vi "XBOX_Joystick_Name.vi"(9 "POVs":i16[](array[numeric]), 10 "Buttons":bool[](array[boolean]), 11 "Axes":dbl[](array[numeric])) -> (2 "Named Axes":T1, 3 "Named Buttons":T2)   [LabVIEW 2018]
uses:
  TypeDefs/XBoxButtons_Type.ctl
  TypeDefs/XBoxAxes_Type.ctl
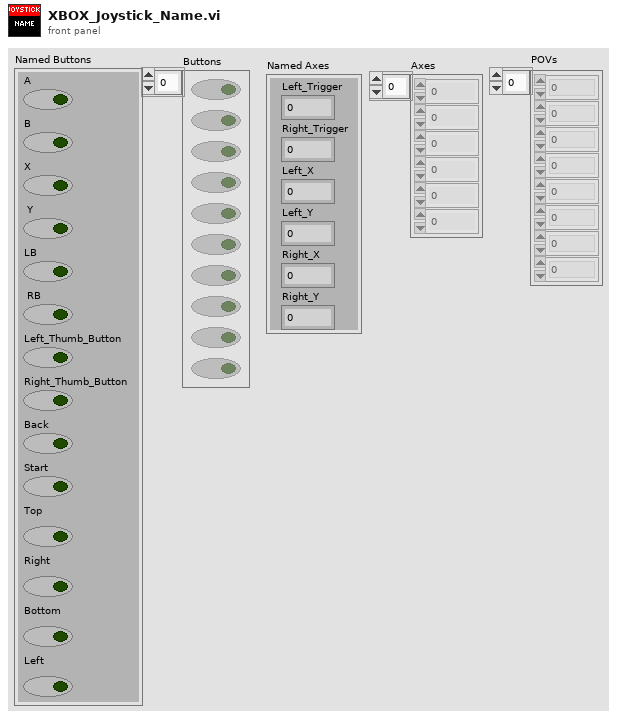
[diagram p1: front panel]
types:
  T1 = typedef "XBoxAxes_Type.ctl" = cluster{"Left_Trigger":dbl, "Right_Trigger ":dbl, "Left_X":dbl, "Left_Y":dbl, "Right_X":dbl, "Right_Y":dbl}
  T2 = typedef "XBoxButtons_Type.ctl" = cluster{"A":bool, "B":bool, "X":bool, " Y":bool, "LB":bool, " RB":bool, "Left_Thumb_Button":bool, "Right_Thumb_Button":bool, "Back":bool, "Start":bool, "Top":bool, "Right":bool, "Bottom":bool, "Left":bool}
  T3 = cluster{"Axes[0]":dbl, "Axes[1]":dbl, "Axes[2]":dbl, "Axes[3]":dbl, "Axes[4]":dbl, "Axes[5]":dbl}
  T4 = cluster{"Buttons[0]":bool, "Buttons[1]":bool, "Buttons[2]":bool, "Buttons[3]":bool, "Buttons[4]":bool, "Buttons[5]":bool, "Buttons[6]":bool, "Buttons[7]":bool, "Buttons[8]":bool, "Buttons[9]":bool}
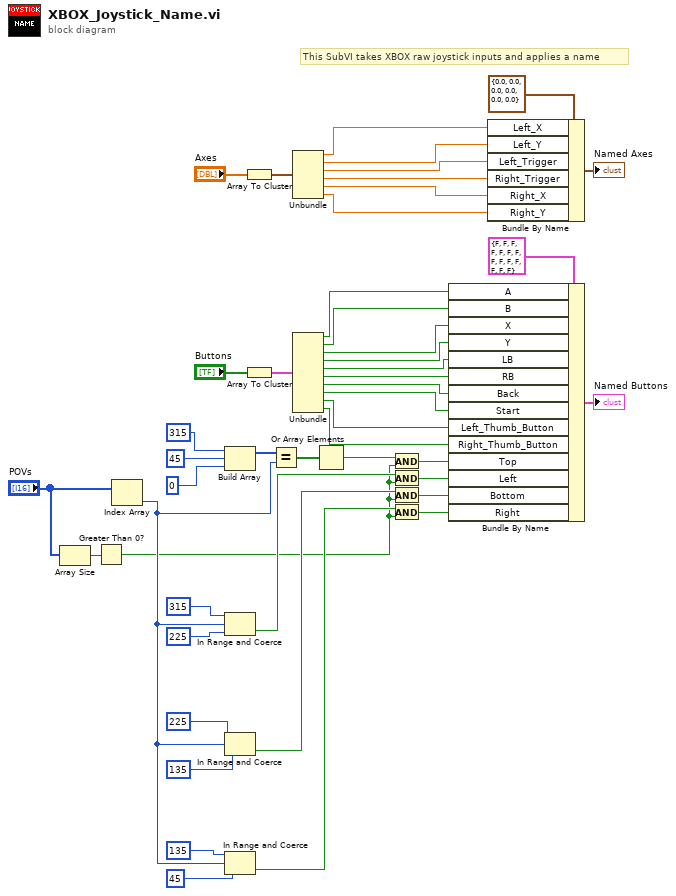
[diagram p0: block diagram]
diagram:
  # "This SubVI takes XBOX raw joystick inputs and applies a name"
  n1 = Array Size(array="POVs") -> (size(s)=w7:i32)
  n2 = Greater Than 0?(x=w7) -> (x > 0?=w1:bool)
  n3 = Index Array(array="POVs") -> (element=w10:i16)  [unwired: 1 in]
  n4 = Build Array(i16 315 ("upper limit"), i16 45 ("element"), i16 0 ("element")) -> (w11:i16[])
  n5 = In Range and Coerce(upper limit=i16 315, x=w10, lower limit=i16 225) -> (In Range?=w17:bool)  [unwired: 1 out]
  n6 = In Range and Coerce(upper limit=i16 225, x=w10, lower limit=i16 135) -> (In Range?=w16:bool)  [unwired: 1 out]
  n7 = In Range and Coerce(upper limit=i16 135, x=w10, lower limit=i16 45) -> (In Range?=w2:bool)  [unwired: 1 out]
  n8 = Array To Cluster(array="Axes") -> (cluster=w30:T3)
  n9 = Array To Cluster(array="Buttons") -> (cluster=w27:T4)
  n10 = Equal?(x=w11, y=w10) -> (x = y?=w12:bool[])
  n11 = Unbundle(w30) -> ("Axes[0]"=w42:dbl, "Axes[1]"=w43:dbl, "Axes[2]"=w44:dbl, "Axes[3]"=w45:dbl, "Axes[4]"=w46:dbl, "Axes[5]"=w47:dbl)
  n12 = Unbundle(w27) -> ("Buttons[0]"=w32:bool, "Buttons[1]"=w33:bool, "Buttons[2]"=w34:bool, "Buttons[3]"=w35:bool, "Buttons[4]"=w36:bool, "Buttons[5]"=w37:bool, "Buttons[6]"=w38:bool, "Buttons[7]"=w39:bool, "Buttons[8]"=w40:bool, "Buttons[9]"=w26:bool)
  n13 = Or Array Elements(Boolean array=w12) -> (logical OR=w9:bool)
  n14 = And(x=w9, y=w1) -> (x .and. y?=w6:bool)
  n15 = And(x=w17, y=w1) -> (x .and. y?=w5:bool)
  n16 = And(x=w16, y=w1) -> (x .and. y?=w4:bool)
  n17 = And(x=w2, y=w1) -> (x .and. y?=w3:bool)
  n18 = Bundle By Name(cluster=T2 {"A"=FALSE, "B"=FALSE, "X"=FALSE, " Y"=FALSE, "LB"=FALSE, " RB"=FALSE, "Left_Thumb_Button"=FALSE, "Right_Thumb_Button"=FALSE, "Back"=FALSE, "Start"=FALSE, "Top"=FALSE, "Right"=FALSE, "Bottom"=FALSE, "Left"=FALSE}, "A"=w32, "B"=w33, "X"=w34, "Y"=w35, "LB"=w36, "RB"=w37, "Back"=w38, "Start"=w39, "Left_Thumb_Button"=w40, "Right_Thumb_Button"=w26, "Top"=w6, "Left"=w5, "Bottom"=w4, "Right"=w3) -> (→"Named Buttons":T2)
  n19 = Bundle By Name(cluster=T1 {"Left_Trigger"=0.0, "Right_Trigger "=0.0, "Left_X"=0.0, "Left_Y"=0.0, "Right_X"=0.0, "Right_Y"=0.0}, "Left_X"=w42, "Left_Y"=w43, "Left_Trigger"=w44, "Right_Trigger"=w45, "Right_X"=w46, "Right_Y"=w47) -> (→"Named Axes":T1)
